vi "Bidirectional Quadrature Decoder with reset.vi"(9 "Reset":bool, 10 "B":bool, 11 "A":bool) -> (3 "Counter":i32)   [LabVIEW 2017]
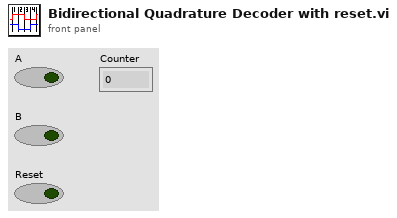
[diagram p1: front panel]
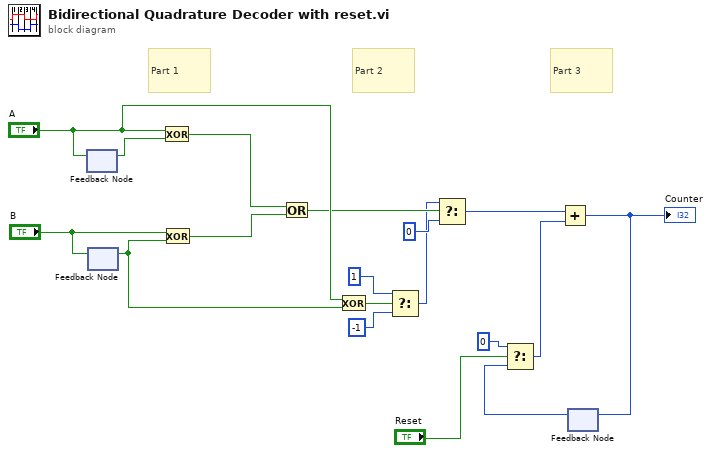
[diagram p0: block diagram]
diagram:
  # "Part 3"
  # "Part 2"
  # "Part 1"
  n1 = feedback #1() -> (w13:bool)  [unwired: 1 in]
  n2 = feedback-in #1("A") -> ()
  n3 = feedback #2() -> (w15:bool)  [unwired: 1 in]
  n4 = feedback-in #2("B") -> ()
  n5 = Exclusive Or(1:w13, 2:"A") -> (0:w11:bool)
  n6 = Exclusive Or(1:w15, 2:"B") -> (0:w6:bool)
  n7 = Or(x=w11, y=w6) -> (x .or. y?=w7:bool)
  n8 = Exclusive Or(1:w15, 2:"A") -> (0:w5:bool)
  n9 = Select(t=1, s=w5, f=-1) -> (s? t:f=w2:i32)
  n10 = Select(t=w2, s=w7, f=0) -> (s? t:f=w9:i32)
  n11 = feedback #3() -> (w16:i32)  [unwired: 1 in]
  n12 = Select(t=0, s="Reset", f=w16) -> (s? t:f=w18:i32)
  n13 = Add(x=w9, y=w18) -> (x+y=w8:i32)
  "Counter" <- w8
  n14 = feedback-in #3(w8) -> ()
